vi "MakeErrorObsolete.vi"(8 "ErrorIn":errorcluster caption="Error In(no Error)", 10 "ErrorCode":i32, 11 "ReferenceIn":refnum<class "ErrorDefinitionSQLite.lvclass"> caption="Reference In") -> (0 "ErrorOut":errorcluster caption="Error Out", 3 "ReferenceOut":refnum<class "ErrorDefinitionSQLite.lvclass"> caption="Reference Out")   [LabVIEW 2018, in "ErrorDefinitionSQLite.lvclass"]
uses:
  <userlib>/_express/CustomErrorCreator/ErrorDefinitionSQLite/ErrorDefinitionSQLite.lvclass
  <vilib>/drjdpowell/SQLite Library/SQL Connection/Open (path).vi
  <vilib>/drjdpowell/SQLite Library/SQL Connection/Open (string).vi
  <vilib>/AdvancedString/Path To Command Line String.vi
  <vilib>/drjdpowell/SQLite Library/SQL Connection/Execute SQL.vi
  <vilib>/drjdpowell/SQLite Library/SQL Connection/Connection.lvclass
  <vilib>/drjdpowell/SQLite Library/SQLite.lvlib
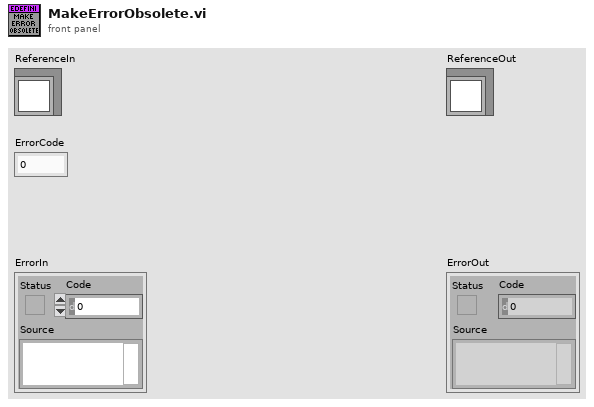
[diagram p1: front panel]
types:
  T1 = enum16{"New or existing", "Existing", "Read only"}
  T2 = typedef "ErrorDefinitionSQLite.lvclass/ObjectAttributes.ctl" = cluster{"Path":path}
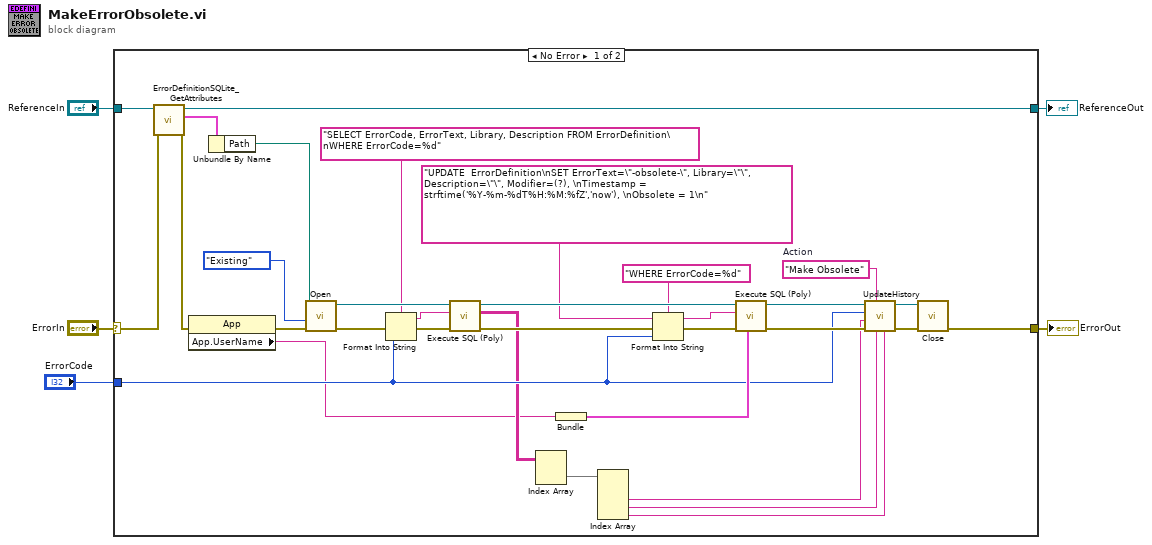
[diagram p0: block diagram]
diagram:
  n1 = case shown="No Error" "ErrorIn" {
    selector: "ErrorIn" -> [w38 w40]
    tunnel: [w32 w40] -> w4
    tunnel: [w36 w39] -> w2
    tunnel: "ReferenceIn" -> [w37 w39]
    tunnel: "ErrorCode" -> [w17 _]
    frame No Error {
      w28 = "Make Obsolete"  # Action
      n2 = call <userlib>:"ErrorDefinitionSQLite_GetAttributes.vi"("ErrorIn"=w38, "Reference in"=w37) -> ("ErrorOut"=w10:errorcluster, "Data"=w34:T2, "Reference out"=w36:refnum<class "ErrorDefinitionSQLite.lvclass">)  [unwired: 6 in, 1 out]
      n3 = property class="App"(error in=w10) -> (error out=w9:errorcluster, "App.UserName"=w6:string)  [unwired: 1 in, 1 out]
      n4 = Unbundle By Name(w34) -> ("Path"=w33:path)
      n5 = call-poly <vilib>:"Open.vi"("error in (no error)"=w9, "File Option"=T1."Existing", "db file"=w33) -> ("error out"=w19:errorcluster, "SQLite Connection"=w23:refnum<class "Connection.lvclass">)  [unwired: 7 in]
      n6 = Format Into String(format string="SELECT ErrorCode, ErrorText, Library, Description FROM ErrorDefinition\nWHERE ErrorCode=%d" ("SQL"), error in=w19, w17) -> (resulting string=w16:string, error out=w18:errorcluster)  [unwired: 1 in]
      n7 = call-poly <vilib>:"Execute SQL (Poly).vi"("error in (no error)"=w18, "SQL"=w16, "SQLite Connection in"=w23) -> ("error out"=w22:errorcluster, "Result Set"=w15:string[][], "SQLite Connection"=w21:refnum<class "Connection.lvclass">)  [unwired: 5 in, 1 out]
      n8 = Index Array(array=w15) -> (element=w14:string[])  [unwired: 2 in]
      n9 = Bundle("App.UserName"=w6) -> (w29:cluster{"App.UserName":string})  [unwired: 1 in]
      n10 = Index Array(array=w14) -> (element #2=w13:string, element #3=w12:string, element #4=w11:string)  [unwired: 4 in, 1 out]
      n11 = Format Into String(format string="WHERE ErrorCode=%d" ("SQL"), initial string="UPDATE  ErrorDefinition\nSET ErrorText=\"-obsolete-\", Library=\"\", Description=\"\", Modifier=(?), \nTimestamp = strftime('%Y-%m-%dT%H:%M:%fZ','now'), \nObsolete = 1\n" ("SQL"), error in=w22, w17) -> (resulting string=w30:string, error out=w31:errorcluster)
      n12 = call-poly <vilib>:"Execute SQL (Poly).vi"("Parameter(s)"=w29, "error in (no error)"=w31, "SQL"=w30, "SQLite Connection in"=w21) -> ("error out"=w24:errorcluster, "SQLite Connection"=w27:refnum<class "Connection.lvclass">)  [unwired: 4 in, 2 out]
      n13 = call <userlib>:"UpdateHistory.vi"("Description"=w11, "Library"=w12, "Action"=w28, "error in (no error)"=w24, "ErrorText"=w13, "ErrorCode"=w17, "Connection in"=w27) -> ("error out"=w25:errorcluster, "Connection out"=w26:refnum<class "Connection.lvclass">)  [unwired: 3 in]
      n14 = call-dynamic "Close.vi"("error in (no error)"=w25, "SQLite Connection in"=w26) -> ("error out"=w32:errorcluster)  [unwired: 9 in]
    }
    frame Error {
    }
  }
  "ErrorOut" <- w4
  "ReferenceOut" <- w2
